vi "Template Test.vi"(0 "Shape":T1, 1 "Sample Frequency":dbl, 2 "Sample Count":dbl, 5 "Frequency":T2, 7 "Amplitude":T2, 9 "Phase":T2, 11 "Offset":T2) -> (4 "Out":T3)   [LabVIEW 2020]
uses:
  <extravilib>/ChannelInstances/Flex-c(dbl,dbl,a[.](dbl))/))Channel.ctl
  <extravilib>/ChannelInstances/Flex-dbl/))Channel.ctl
  <extravilib>/ChannelInstances/Flex-t'Function Generator.lvlib-Shape.ctl'/))Channel.ctl
  FlexBlocks/Shape.ctl
  Workers/Function Generator/State.ctl
  FlexBlocks/Block State.ctl
  FlexBlocks/Command.ctl
  Workers/Function Generator/Init.ctl
  FlexBlocks/Worker Action.ctl
  Workers/Function Generator/Tags.ctl
  Workers/Function Generator/Work.vi
  FlexBlocks/FlexBlocks.lvlib
  <extravilib>/ChannelInstances/Flex-c(dbl,dbl,a[.](dbl)).lvlib
  Workers/Function Generator/Function Generator.lvlib
  <extravilib>/ChannelInstances/Flex-dbl.lvlib
  <extravilib>/ChannelInstances/Flex-t'Function Generator.lvlib-Shape.ctl'.lvlib
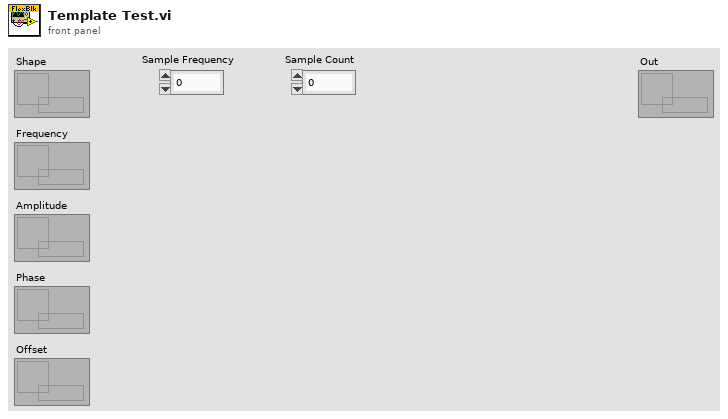
[diagram p1: front panel]
types:
  T1 = typedef "Flex-t'Function Generator.lvlib-Shape.ctl'.lvlib/))Channel.ctl" = refnum<queue>
  T2 = typedef "Flex-dbl.lvlib/))Channel.ctl" = refnum<queue>
  T3 = typedef "Flex-c(dbl,dbl,a[.](dbl)).lvlib/))Channel.ctl" = refnum<queue>
  T4 = typedef "FlexBlocks.lvlib/Block State.ctl" = enum16{"Idle", "Init", "Start", "Run", "Stop"}
  T5 = typedef "Function Generator.lvlib/State.ctl" = cluster{"dt":dbl}
  T6 = typedef "FlexBlocks.lvlib/Command.ctl" = enum16{"Close", "Step", "Run", "Pause", "Init"}
  T7 = typedef "FlexBlocks.lvlib/Worker Action.ctl" = enum16{"Start", "Work", "Stop"}
  T8 = typedef "Function Generator.lvlib/Tags.ctl" = cluster{"Shape":T9, "Frequency":dbl, "Amplitude":dbl, "Phase":dbl, "Offset":dbl}
  T9 = typedef "Function Generator.lvlib/Shape.ctl" = enum16{"Sine", "Square", "Triangle", "Saw"}
  T10 = typedef "FlexBlocks.lvlib/Block Status.ctl" = cluster{"State":T4, "i":i32, "Init":bool, "Started":bool, "Action":T11}
  T11 = typedef "FlexBlocks.lvlib/Run Action.ctl" = enum16{"N/A", "Read", "Work", "Write"}
  T12 = typedef "Function Generator.lvlib/Init.ctl" = cluster{"Sample Frequency":dbl, "Sample Count":dbl}
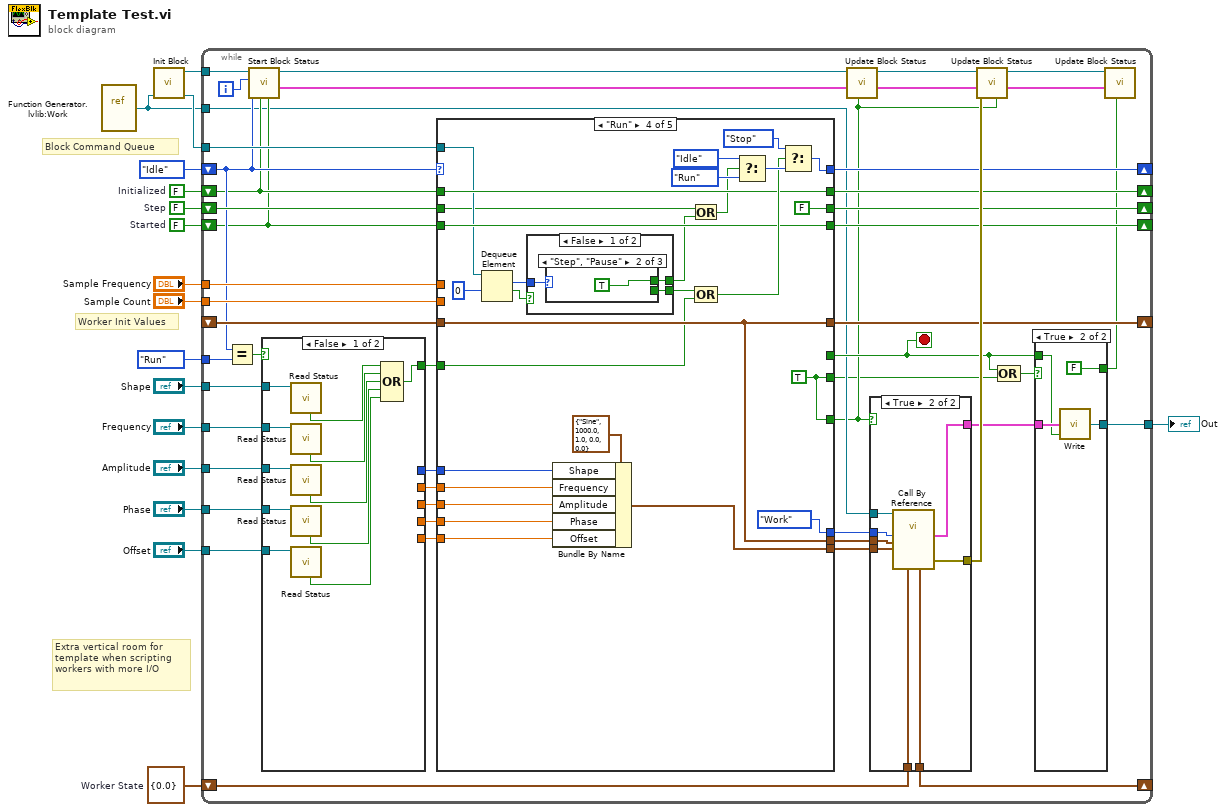
[diagram p0: block diagram]
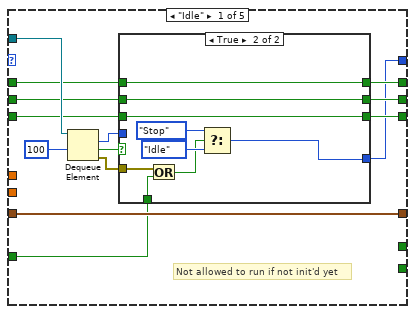
[diagram p2: hidden frame]
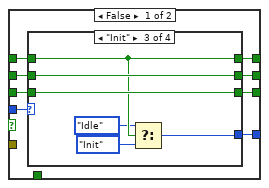
[diagram p3: hidden frame]
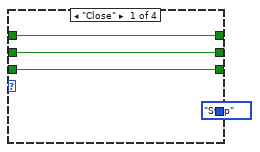
[diagram p4: hidden frame]
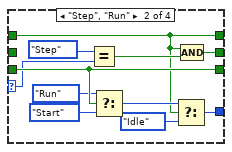
[diagram p5: hidden frame]
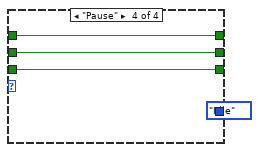
[diagram p6: hidden frame]
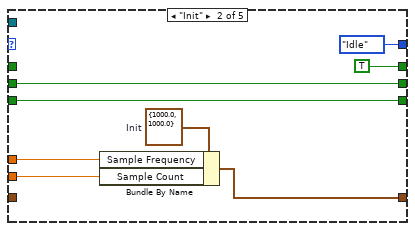
[diagram p7: hidden frame]
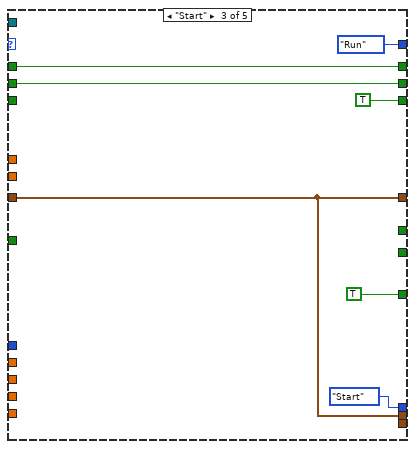
[diagram p8: hidden frame]
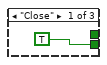
[diagram p9: hidden frame]
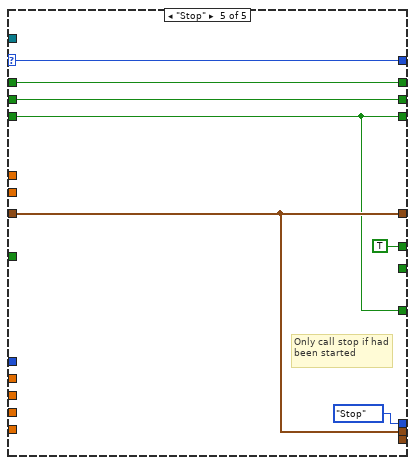
[diagram p12: hidden frame]
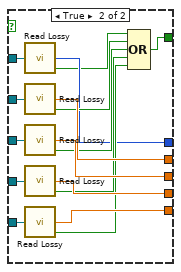
[diagram p13: hidden frame]
diagram:
  w6 = FALSE  # Initialized
  w7 = FALSE  # Step
  w8 = FALSE  # Started
  w17 = T5 {"dt"=0.0}  # Worker State
  # "Extra vertical room for template when scripting workers with more I/O"
  # "Block Command Queue"
  # "Worker Init Values"
  n1 = vi-ref "Function Generator.lvlib:Work.vi"() -> (w2:refnum<vi>)
  n2 = call "Init Block.vi"("Worker VI"=w2) -> ("Command Queue"=w5:refnum<queue>, "Status Queue"=w4:refnum<queue>)  [unwired: 9 in]
  n3 = while {
    shift-right: [w22] -> _
    shift-left: w17 -> [w23]
    shift-right: [w54] -> _
    shift-left: Block_State."Idle" ("Block State") -> [w35]
    tunnel: [w51] -> w15
    shift-right: [w63] -> _
    shift-left: _ -> [w62]
    tunnel: "Frequency" -> [w49]
    tunnel: "Amplitude" -> [w48]
    tunnel: "Phase" -> [w47]
    tunnel: "Offset" -> [w46]
    tunnel: "Sample Frequency" -> [w60]
    tunnel: "Sample Count" -> [w59]
    shift-right: [w52] -> _
    shift-left: w8 -> [w33]
    shift-right: [w56] -> _
    shift-left: w7 -> [w58]
    shift-right: [w53] -> _
    shift-left: w6 -> [w34]
    tunnel: w5 -> [w55]
    tunnel: w4 -> [w37]
    tunnel: Block_State."Run" ("Block State") -> [w40]
    tunnel: w2 -> [w24]
    tunnel: "Shape" -> [w21]
    i -> [w36]
    stop <- w25 stop-if-true
    n4 = Equal?(x=w35, y=w40) -> (x = y?=w39:bool)
    n5 = call "Start Block Status.vi"("Started"=w33, "Init"=w34, "Block State"=w35, "i"=w36, "Status Queue In"=w37) -> ("Status"=w31:T10, "Status Queue"=w32:refnum<queue>)  [unwired: 5 in]
    n6 = case shown="False" w39 {
      tunnel: w49 -> [w187 w203]
      tunnel: w48 -> [w184 w202]
      tunnel: w47 -> [w185 w201]
      tunnel: w46 -> [w186 w200]
      tunnel: [_ w190] -> w45
      tunnel: [_ w199] -> w44
      tunnel: [_ w198] -> w43
      tunnel: [_ w197] -> w42
      tunnel: [_ w196] -> w41
      tunnel: [w183 w195] -> w38
      tunnel: w21 -> [w178 w188]
      frame False {
        n7 = call <extravilib>:"Read Status.vi"("channel"=w178) -> ("Closed?"=w177:bool)  [unwired: 4 in, 6 out]
        n8 = call <extravilib>:"Read Status.vi"("channel"=w187) -> ("Closed?"=w182:bool)  [unwired: 4 in, 6 out]
        n9 = call <extravilib>:"Read Status.vi"("channel"=w184) -> ("Closed?"=w181:bool)  [unwired: 4 in, 6 out]
        n10 = call <extravilib>:"Read Status.vi"("channel"=w185) -> ("Closed?"=w180:bool)  [unwired: 4 in, 6 out]
        n11 = call <extravilib>:"Read Status.vi"("channel"=w186) -> ("Closed?"=w179:bool)  [unwired: 4 in, 6 out]
        n12 = Compound Arithmetic op=OR(w177, w182, w181, w180, w179) -> (w183:bool)
      }
      frame True {
        n13 = call <extravilib>:"Read Lossy.vi"("FlexChannel"=w188) -> ("Value"=w190:T9, "Closed?"=w189:bool)  [unwired: 2 in, 3 out]
        n14 = call <extravilib>:"Read Lossy.vi"("FlexChannel"=w203) -> ("Value"=w199:dbl, "Closed?"=w194:bool)  [unwired: 2 in, 3 out]
        n15 = call <extravilib>:"Read Lossy.vi"("FlexChannel"=w202) -> ("Value"=w198:dbl, "Closed?"=w193:bool)  [unwired: 2 in, 3 out]
        n16 = call <extravilib>:"Read Lossy.vi"("FlexChannel"=w201) -> ("Value"=w197:dbl, "Closed?"=w192:bool)  [unwired: 2 in, 3 out]
        n17 = call <extravilib>:"Read Lossy.vi"("FlexChannel"=w200) -> ("Value"=w196:dbl, "Closed?"=w191:bool)  [unwired: 2 in, 3 out]
        n18 = Compound Arithmetic op=OR(w189, w194, w193, w192, w191) -> (w195:bool)
      }
    }
    n19 = case shown="\"Run\"" w35 {
      selector: w35 -> [_ _ _ _ w171]
      tunnel: [_ _ w133 w162 w176] -> w64
      tunnel: [w79 w122 w133 w162 w176] -> w63
      tunnel: [_ _ TRUE w137 w173] -> w20
      tunnel: w62 -> [w79 _ w133 w162 w176]
      tunnel: [_ _ _ w163 _] -> w61
      tunnel: w60 -> [_ w128 _ _ _]
      tunnel: w59 -> [_ w127 _ _ _]
      tunnel: [w67 Block_State."Idle" ("Block State") Block_State."Run" ("Block State") w159 w171] -> w54
      tunnel: w33 -> [w71 w124 _ w155 w173]
      tunnel: w58 -> [w72 w123 w132 w148 w170]
      tunnel: [_ _ Worker_Action."Start" ("State") Worker_Action."Work" ("State") Worker_Action."Stop" ("State")] -> w57
      tunnel: [_ _ _ _ TRUE] -> w25
      tunnel: [w69 w123 w132 FALSE ("Step") w170] -> w56
      tunnel: [w70 w124 TRUE ("Started") w155 w173] -> w52
      tunnel: w34 -> [w73 _ w131 w156 w172]
      tunnel: [w68 TRUE ("Initialized") w131 w156 w172] -> w53
      tunnel: w55 -> [w77 _ _ w154 _]
      tunnel: w45 -> [_ _ _ w138 _]
      tunnel: w44 -> [_ _ _ w143 _]
      tunnel: w43 -> [_ _ _ w142 _]
      tunnel: w42 -> [_ _ _ w141 _]
      tunnel: w41 -> [_ _ _ w140 _]
      tunnel: w38 -> [w66 _ _ w139 _]
      tunnel: [_ _ _ w137 _] -> w19
      frame "Idle" {
        # "Not allowed to run if not init'd yet"
        n20 = Dequeue Element(queue=w77, timeout in ms (-1)=100) -> (element=w76:T6, timed out?=w75:bool, error out=w74:errorcluster)  [unwired: 1 in, 1 out]
        n21 = case shown="True" w75 {
          tunnel: w76 -> [w87 _]
          tunnel: w74 -> [_ w115]
          tunnel: [w83 w119] -> w67
          tunnel: w73 -> [w86 w116]
          tunnel: w72 -> [w85 w117]
          tunnel: w71 -> [w84 w118]
          tunnel: [w80 w118] -> w70
          tunnel: [w81 w117] -> w69
          tunnel: [w82 w116] -> w68
          tunnel: w66 -> [_ w114]
          frame False {
            n22 = case shown="\"Init\"" w87 {
              selector: w87 -> [_ w96 _ _]
              tunnel: w86 -> [w91 w92 w106 w111]
              tunnel: w85 -> [w90 _ w108 w110]
              tunnel: w84 -> [w89 w98 w107 w109]
              tunnel: [Block_State."Stop" ("Block State") w102 w104 Block_State."Idle" ("Block State")] -> w83
              tunnel: [w91 w92 w106 w111] -> w82
              tunnel: [w90 w93 w108 w110] -> w81
              tunnel: [w89 w98 w107 w109] -> w80
              frame "Close" {
              }
              frame "Step", "Run" {
                n23 = Equal?(x=Command."Step" ("y"), y=w96) -> (x = y?=w94:bool)
                n24 = Select(t=Block_State."Run", s=w98, f=Block_State."Start" ("Block State")) -> (s? t:f=w100:T4)
                n25 = Select(t=w100, s=w92, f=Block_State."Idle" ("Block State")) -> (s? t:f=w102:T4)
                n26 = Compound Arithmetic op=AND(w92, w94) -> (w93:bool)
              }
              frame "Init" {
                n27 = Select(t=Block_State."Idle" ("Block State"), s=w106, f=Block_State."Init" ("Block State")) -> (s? t:f=w104:T4)
              }
              frame "Pause" {
              }
            }
          }
          frame True {
            n28 = Or(x=w115, y=w114) -> (x .or. y?=w113:bool)
            n29 = Select(t=Block_State."Stop" ("Block State"), s=w113, f=Block_State."Idle" ("Block State")) -> (s? t:f=w119:T4)
          }
        }
      }
      frame "Init" {
        w129 = T12 {"Sample Frequency"=1000.0, "Sample Count"=1000.0}  # Init
        n30 = Bundle By Name(cluster=w129, "Sample Frequency"=w128, "Sample Count"=w127) -> (w122:T12)
      }
      frame "Start" {
      }
      frame "Run" {
        w137 = TRUE
        n31 = Dequeue Element(queue=w154, timeout in ms (-1)=0) -> (element=w152:T6, timed out?=w151:bool)  [unwired: 1 in, 2 out]
        n32 = case shown="False" w151 {
          tunnel: w152 -> [w167 _]
          tunnel: [w166 _] -> w150
          tunnel: [w165 _] -> w146
          frame False {
            n33 = case shown="\"Step\", \"Pause\"" w167 {
              tunnel: [_ TRUE _] -> w165
              tunnel: [TRUE _ _] -> w166
              frame "Close" {
              }
              frame "Step", "Pause" {
              }
              frame "Run", "Init" {
              }
            }
          }
          frame True {
          }
        }
        n34 = Bundle By Name(cluster=T8 {"Shape"=enum."Sine", "Frequency"=1000.0, "Amplitude"=1.0, "Phase"=0.0, "Offset"=0.0} ("Tags"), "Shape"=w138, "Frequency"=w143, "Amplitude"=w142, "Phase"=w141, "Offset"=w140) -> (w163:T8)
        n35 = Or(x=w148, y=w146) -> (x .or. y?=w145:bool)
        n36 = Compound Arithmetic op=OR(w150, w139) -> (w158:bool)
        n37 = Select(t=Block_State."Idle" ("Block State"), s=w145, f=Block_State."Run" ("Block State")) -> (s? t:f=w160:T4)
        n38 = Select(t=Block_State."Stop", s=w158, f=w160) -> (s? t:f=w159:T4)
      }
      frame "Stop" {
        # "Only call stop if had been started"
      }
    }
    n39 = call "Update Block Status.vi"("Working"=w20, "Status In"=w31, "Status Queue In"=w32) -> ("Status"=w27:T10, "Status Queue"=w30:refnum<queue>)  [unwired: 7 in]
    n40 = case shown="True" w20 {
      tunnel: w64 -> [_ w210]
      tunnel: w61 -> [_ w209]
      tunnel: w57 -> [_ w211]
      tunnel: [_ w208] -> w50
      tunnel: w24 -> [_ w212]
      tunnel: w23 -> [w204 w207]
      tunnel: [w204 w206] -> w22
      tunnel: [_ w205] -> w65
      frame False {
      }
      frame True {
        n41 = call-by-ref "?"(reference=w212, "State"=w211, "Init"=w210, "Tags"=w209, "State in"=w207) -> ("Out"=w208:cluster{"t0":dbl, "dt":dbl, "y":dbl[]}, "State out"=w206:T5, "error out"=w205:errorcluster)  [unwired: 10 in, 2 out]
      }
    }
    n42 = call "Update Block Status.vi"("Writing"=w20, "Worker Error"=w65, "Status In"=w27, "Status Queue In"=w30) -> ("Status"=w28:T10, "Status Queue"=w29:refnum<queue>)  [unwired: 6 in]
    n43 = Compound Arithmetic op=OR(w25, w19) -> (w18:bool)
    n44 = case shown="True" w18 {
      tunnel: w50 -> [_ w216]
      tunnel: [_ w215] -> w51
      tunnel: w25 -> [_ w214]
      tunnel: [_ FALSE ("Writing")] -> w26
      frame False {
      }
      frame True {
        n45 = call <extravilib>:"Write.vi"("element"=w216, "Close? (F)"=w214) -> ("channel"=w215:T3)  [unwired: 3 in, 2 out]
      }
    }
    n46 = call "Update Block Status.vi"("Working"=w26, "Status In"=w28, "Status Queue In"=w29) -> ()  [unwired: 7 in, 2 out]
  }
  "Out" <- w15
